vi "Read Last Switch.vi"(8 "error in (no error)":errorcluster, 11 "Output Timer in":refnum<class "Output Timer.lvclass">) -> (0 "error out":errorcluster, 2 "Last Switch":timestamp format="%<%H:%M:%S%2u>T", 3 "Output Timer out":refnum<class "Output Timer.lvclass">)   [LabVIEW 2013, in "Output Timer.lvclass"]
uses:
  Output Timer.lvclass
  Output Timer.lvclass/Output Timer.ctl
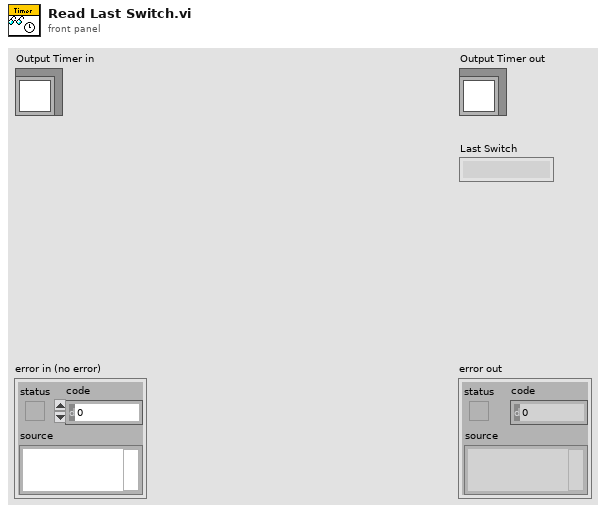
[diagram p1: front panel]
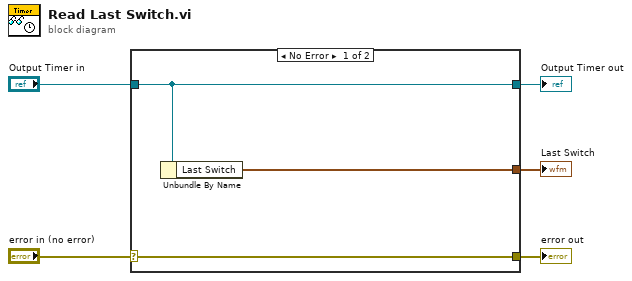
[diagram p0: block diagram]
diagram:
  n1 = case shown="No Error" "error in (no error)" {
    selector: "error in (no error)" -> [w8 w9]
    tunnel: [w8 w9] -> w4
    tunnel: [w7 w10] -> w2
    tunnel: "Output Timer in" -> [w7 w10]
    tunnel: [w6 _] -> w1
    frame No Error {
      n2 = Unbundle By Name(w7) -> ("Last Switch"=w6:timestamp)
    }
    frame Error {
    }
  }
  "error out" <- w4
  "Output Timer out" <- w2
  "Last Switch" <- w1
